vi "Export_Excel.vi"(1 "行首字符串[]":string[](array[string]), 2 "列首字符串[]":string[](array[string]), 3 "table":string[][](table) caption="查询结果") -> ()   [LabVIEW 2014]
uses:
  <vilib>/Utility/file.llb/Write To Spreadsheet File (string).vi
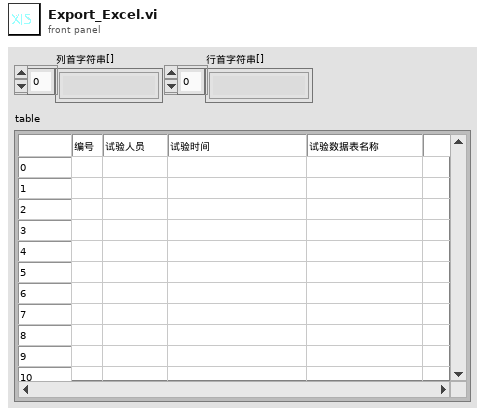
[diagram p1: front panel]
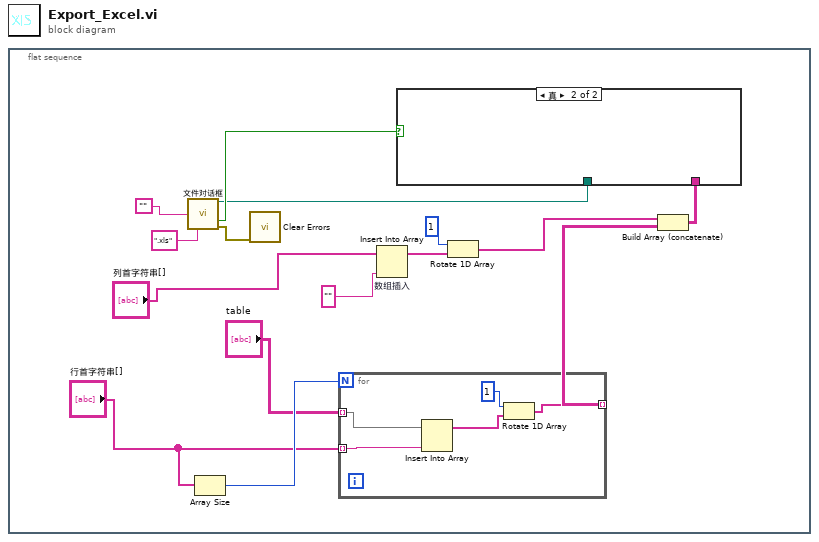
[diagram p0: block diagram]
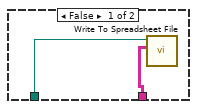
[diagram p2: hidden frame]
diagram:
  n1 = flat-sequence {
    frame #0 {
      n2 = call "文件对话框"("default name"="", "pattern (all files)"=".xls") -> ("selected path"=w7:path, "cancelled"=w8:bool, "error out"=w2:errorcluster)  [unwired: 10 in, 1 out]
      n3 = Array Size(array="行首字符串[]") -> (size(s)=w14:i32)
      n4 = call <vilib>:"Clear Errors.vi"("error in (no error)"=w2) -> ()  [unwired: 5 in, 2 out]
      n5 = for {
        N: w14 -> [_]
        tunnel: "行首字符串[]" -> [w21] mode=indexing
        tunnel: "table" -> [w22] mode=indexing
        tunnel: [w19] -> w13 mode=indexing
        n6 = Insert Into Array(array=w22, new element=w21) -> (w20:string[])  [unwired: 1 in]
        n7 = Rotate 1D Array ("一维数组循环移位")(1:w20, 2:1 ("n")) -> (0:w19:string[])
      }
      n8 = Insert Into Array "数组插入"(array="列首字符串[]", new element="" ("新元素/子数组")) -> (w11:string[])  [unwired: 1 in]
      n9 = Rotate 1D Array ("一维数组循环移位")(1:w11, 2:1 ("n")) -> (0:w9:string[])
      n10 = Build Array (concatenate)(w9, w13) -> (w6:string[][])
      n11 = case shown="真" w8 {
        tunnel: w7 -> [w17 _]
        tunnel: w6 -> [w16 _]
        frame False {
          n12 = call-poly <vilib>:"Write To Spreadsheet File.vi"("2D data"=w16, "file path (dialog if empty)"=w17) -> ()  [unwired: 6 in, 1 out]
        }
        frame True {
        }
      }
    }
  }
